vi "Guide.vi"() -> ()   [LabVIEW 2016]
uses:
  Gates/Polymorph/Xtarget.vi
panel:
  out "State vector":cdb[](array[numeric]) format="%#_3g"
  out "Classical bit 1":bool
  out "Classical bit 0":bool
  # "Hello Quantum World!"
  # "Please open the block diagram from the menu bar or press Ctrl+E"
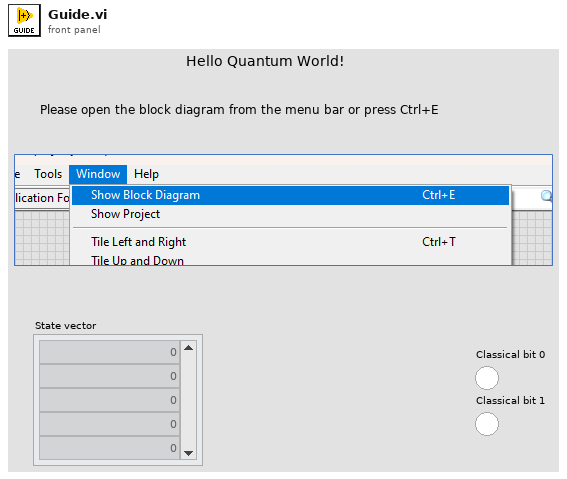
[diagram p1: front panel]
types:
  T1 = typedef "Circuit Cluster.ctl" = cluster{"Loop No":i32, "Wire":cluster{"No":i32, "Depth":i32, "Hold":i32[][], "Permits":refnum<notifier>}, "Size":refnum<queue>, "Composition":refnum<queue>, "Gate class":refnum<class "GateAbst.lvclass">}
  T2 = typedef "Controls.ctl" = i32[][]
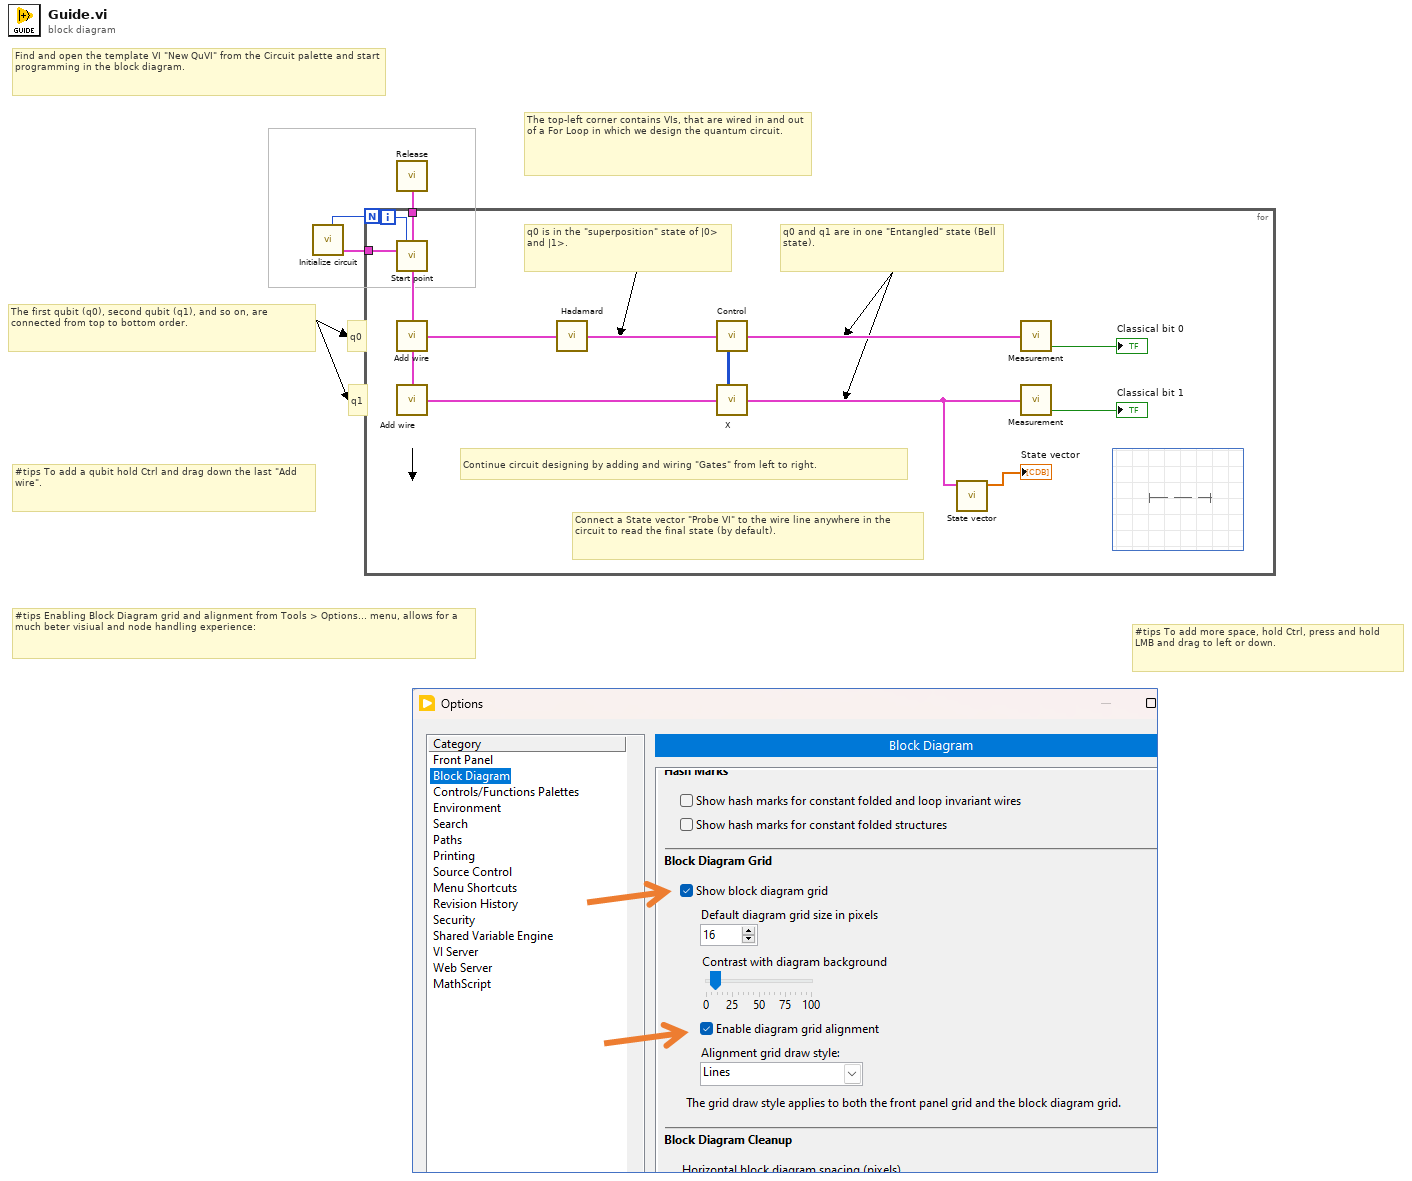
[diagram p0: block diagram]
diagram:
  # "Find and open the template VI \"New QuVI\" from the Circuit palette and start programming in the block diagram."
  # "q1"
  # "q0"
  # "#tips Enabling Block Diagram grid and alignment from Tools > Options... menu, allows for a much beter visiual and node handling experience:"
  # "#tips To add more space, hold Ctrl, press and hold LMB and drag to left or down."
  # "The first qubit (q0), second qubit (q1), and so on, are connected from top to bottom order."
  # "#tips To add a qubit hold Ctrl and drag down the last \"Add wire\"."
  # "The top-left corner contains VIs, that are wired in and out of a For Loop in which we design the quantum circuit."
  n1 = call "Initialize circuit.vi"() -> ("N"=w2:i32, "Circuit cluster"=w3:T1)  [unwired: 8 in]
  n2 = for {
    N: w2 -> [_]
    tunnel: w3 -> [w15]
    tunnel: [w9] -> w1
    i -> [w4]
    # "Connect a State vector \"Probe VI\" to the wire line anywhere in the circuit to read the final state (by default)."
    # "Continue circuit designing by adding and wiring \"Gates\" from left to right."
    # "q0 and q1 are in one \"Entangled\" state (Bell state)."
    # "q0 is in the \"superposition\" state of |0> and |1>."
    n3 = call "Start point.vi"("Loop No"=w4, "Circuit cluster in"=w15) -> ("Up circuit cluster out"=w9:T1, "Down circuit cluster out"=w14:T1)  [unwired: 12 in]
    n4 = call "Add wire.vi"("Circuit cluster in"=w14) -> ("Wire out"=w16:T1, "Circuit cluster out"=w17:T1)  [unwired: 13 in]
    n5 = call "Add wire.vi"("Circuit cluster in"=w17) -> ("Wire out"=w12:T1)  [unwired: 13 in, 1 out]
    n6 = call "Hadamard.vi"("Wire in"=w16) -> ("Wire out"=w13:T1)  [unwired: 4 in]
    n7 = call "Control.vi"("Wire in"=w13) -> ("uc OUT"=w10:T2, "Wire out"=w11:T1)  [unwired: 6 in, 1 out]
    n8 = call-poly "X.vi"("Up control in"=w10, "Wire in"=w12) -> ("Wire out"=w5:T1)  [unwired: 7 in]
    n9 = call "State vector.vi"("Circuit cluster"=w5) -> ("State vector"=→"State vector":cdb[])  [unwired: 10 in]
    n10 = call "Measurement.vi"("Wire in"=w11) -> ("Classical bit"=→"Classical bit 0":bool)  [unwired: 3 in, 1 out]
    n11 = call "Measurement.vi"("Wire in"=w5) -> ("Classical bit"=→"Classical bit 1":bool)  [unwired: 3 in, 1 out]
  }
  n12 = call "Release.vi"("Circuit cluster in"=w1) -> ()  [unwired: 15 in]
